vi "Fetch.vi"(8 "error in (no error)":errorcluster, 9 "Default Value":variant, 10 "Key":string, 11 "Variant in":variant) -> (0 "error out":errorcluster, 1 "Value out":variant, 2 "Found?":bool, 3 "Variant out":variant)   [LabVIEW 2019, in "JSON.lvlib"]
doc: "Fetches <b>Key</b> from the <b>Variant in</b> and returns the <b>Value out</b> . If the key does not exist, this returns the <b>Default Value</b>.\n\nCreated by: Ryan Pacini"
uses:
  JSON.lvlib
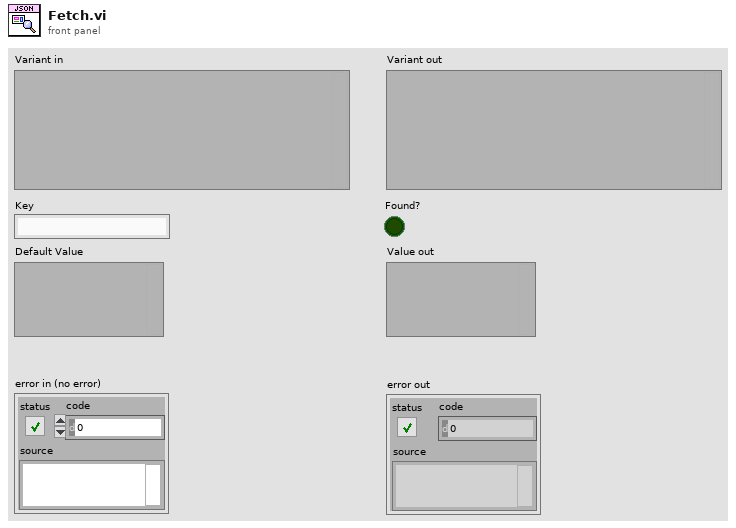
[diagram p1: front panel]
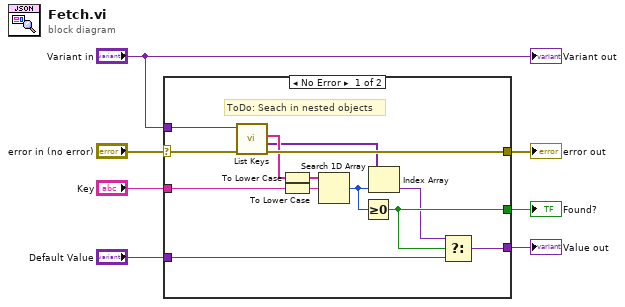
[diagram p0: block diagram]
diagram:
  n1 = case shown="No Error" "error in (no error)" {
    selector: "error in (no error)" -> [w18 w22]
    tunnel: "Default Value" -> [w9 w21]
    tunnel: "Key" -> [w20 _]
    tunnel: [w19 w22] -> w5
    tunnel: "Variant in" -> [w15 _]
    tunnel: [w8 w21] -> w1
    tunnel: [w11 _] -> w2
    frame No Error {
      # "ToDo: Seach in nested objects"
      n2 = call "List Keys.vi"("error in (no error)"=w18, "Variant in"=w15) -> ("error out"=w19:errorcluster, "Values"=w16:variant[], "Keys"=w17:string[])  [unwired: 6 in, 1 out]
      n3 = To Lower Case(string=w17) -> (all lower case string=w14:string[])
      n4 = To Lower Case(string=w20) -> (all lower case string=w13:string)
      n5 = Search 1D Array(1D array=w14, element=w13) -> (index of element=w12:i32)  [unwired: 1 in]
      n6 = Greater Or Equal To 0?(x=w12) -> (x >= 0?=w11:bool)
      n7 = Index Array(array=w16, index=w12) -> (element=w10:variant)
      n8 = Select(t=w10, s=w11, f=w9) -> (s? t:f=w8:variant)
    }
    frame Error {
    }
  }
  "error out" <- w5
  "Found?" <- w2
  "Value out" <- w1
  "Variant out" <- "Variant in"
